vi "test-Coordinate-System-Test5.vi"() -> (3 "All tests passed":bool)   [LabVIEW 2019]
uses:
  <vilib>/Rock Robotics/WPI/ThirdParty/JAS_Junk/TrajLib/VI/CoordAxis_N.vi
  <vilib>/Rock Robotics/WPI/ThirdParty/JAS_Junk/TrajLib/VI/CoordAxis_W.vi
  <vilib>/Rock Robotics/WPI/ThirdParty/JAS_Junk/TrajLib/VI/CoordAxis_U.vi
  <vilib>/Rock Robotics/WPI/ThirdParty/JAS_Junk/TrajLib/VI/CoordSystem_New.vi
  <vilib>/Rock Robotics/WPI/ThirdParty/JAS_Junk/TrajLib/VI/CoordAxis_E.vi
  <vilib>/Rock Robotics/WPI/ThirdParty/JAS_Junk/TrajLib/VI/CoordAxis_D.vi
  <vilib>/Rock Robotics/WPI/ThirdParty/JAS_Junk/TrajLib/Conv_Deg_Radians.vi
  <vilib>/Rock Robotics/WPI/ThirdParty/JAS_Junk/TrajLib/VI/Quaternion_New.vi
  <vilib>/Rock Robotics/WPI/ThirdParty/JAS_Junk/TrajLib/VI/CoordAxis_New.vi
  <vilib>/Rock Robotics/WPI/ThirdParty/JAS_Junk/TrajLib/MatBuilder_Create.vi
  <vilib>/Rock Robotics/WPI/ThirdParty/JAS_Junk/TrajLib/Matrix_AssignBlock.vi
  <vilib>/Rock Robotics/WPI/ThirdParty/JAS_Junk/TrajLib/VI/Rotation3D_Create_RotMatrix.vi
  <vilib>/Rock Robotics/WPI/ThirdParty/JAS_Junk/TrajLib/MatrixHelper_CoerceSize.vi
  <vilib>/Rock Robotics/WPI/ThirdParty/JAS_Junk/TrajLib/VI/Rotation3d_Create_Quaternion.vi
  <vilib>/Rock Robotics/WPI/ThirdParty/JAS_Junk/TrajLib/Matrix_Transpose.vi
  <vilib>/Analysis/baseanly.llb/A x B.vi
  <vilib>/Analysis/baseanly.llb/Real A x B.vi
  <vilib>/Rock Robotics/WPI/ThirdParty/JAS_Junk/TrajLib/Matrix_Ident.vi
  <vilib>/Rock Robotics/WPI/ThirdParty/JAS_Junk/TrajLib/Matrix_IsEqual.vi
  <vilib>/Analysis/baseanly.llb/Determinant.vi
  <vilib>/Analysis/baseanly.llb/Real Determinant.vi
  <vilib>/Rock Robotics/WPI/ThirdParty/JAS_Junk/TrajLib/VI/Quaternion_Normalize.vi
  <vilib>/Rock Robotics/WPI/ThirdParty/JAS_Junk/TrajLib/VI/Quaternion_New_Default.vi
  <vilib>/Analysis/Matrix/Numeric/Conversions/Array To Matrix.vi
  <vilib>/Analysis/Matrix/Numeric/Conversions/Array To Matrix - RA.vi
  <vilib>/Analysis/7linalg.llb/Create Special Matrix.vi
  <vilib>/Analysis/7linalg.llb/Create Special Real Matrix.vi
  <vilib>/Rock Robotics/WPI/ThirdParty/JAS_Junk/TrajLib/Trajectory_Library.lvlib
panel:
  out "Test 4":bool
  out "Test 3":bool
  out "Test 2":bool
  out "Test 1":bool
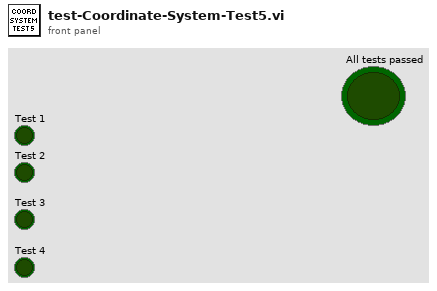
[diagram p1: front panel]
types:
  T1 = typedef "Trajectory_Library.lvlib/TRANSLATION3D.ctl" = cluster{"X":dbl, "Y":dbl, "Z":dbl}
  T2 = typedef "Trajectory_Library.lvlib/ROTATION3D.ctl" = cluster{"Q_quaternion":T3}
  T3 = typedef "Trajectory_Library.lvlib/QUATERNION.ctl" = cluster{"R":dbl, "V":dbl[]}
  T4 = typedef "Trajectory_Library.lvlib/TRANSFORM3D.ctl" = cluster{"TRANSLATION3D":T1, "ROTATION3D":T2, "XF":bool}
  T5 = typedef "Trajectory_Library.lvlib/COORDINATE_SYSTEM.ctl" = cluster{"Rotation":T2}
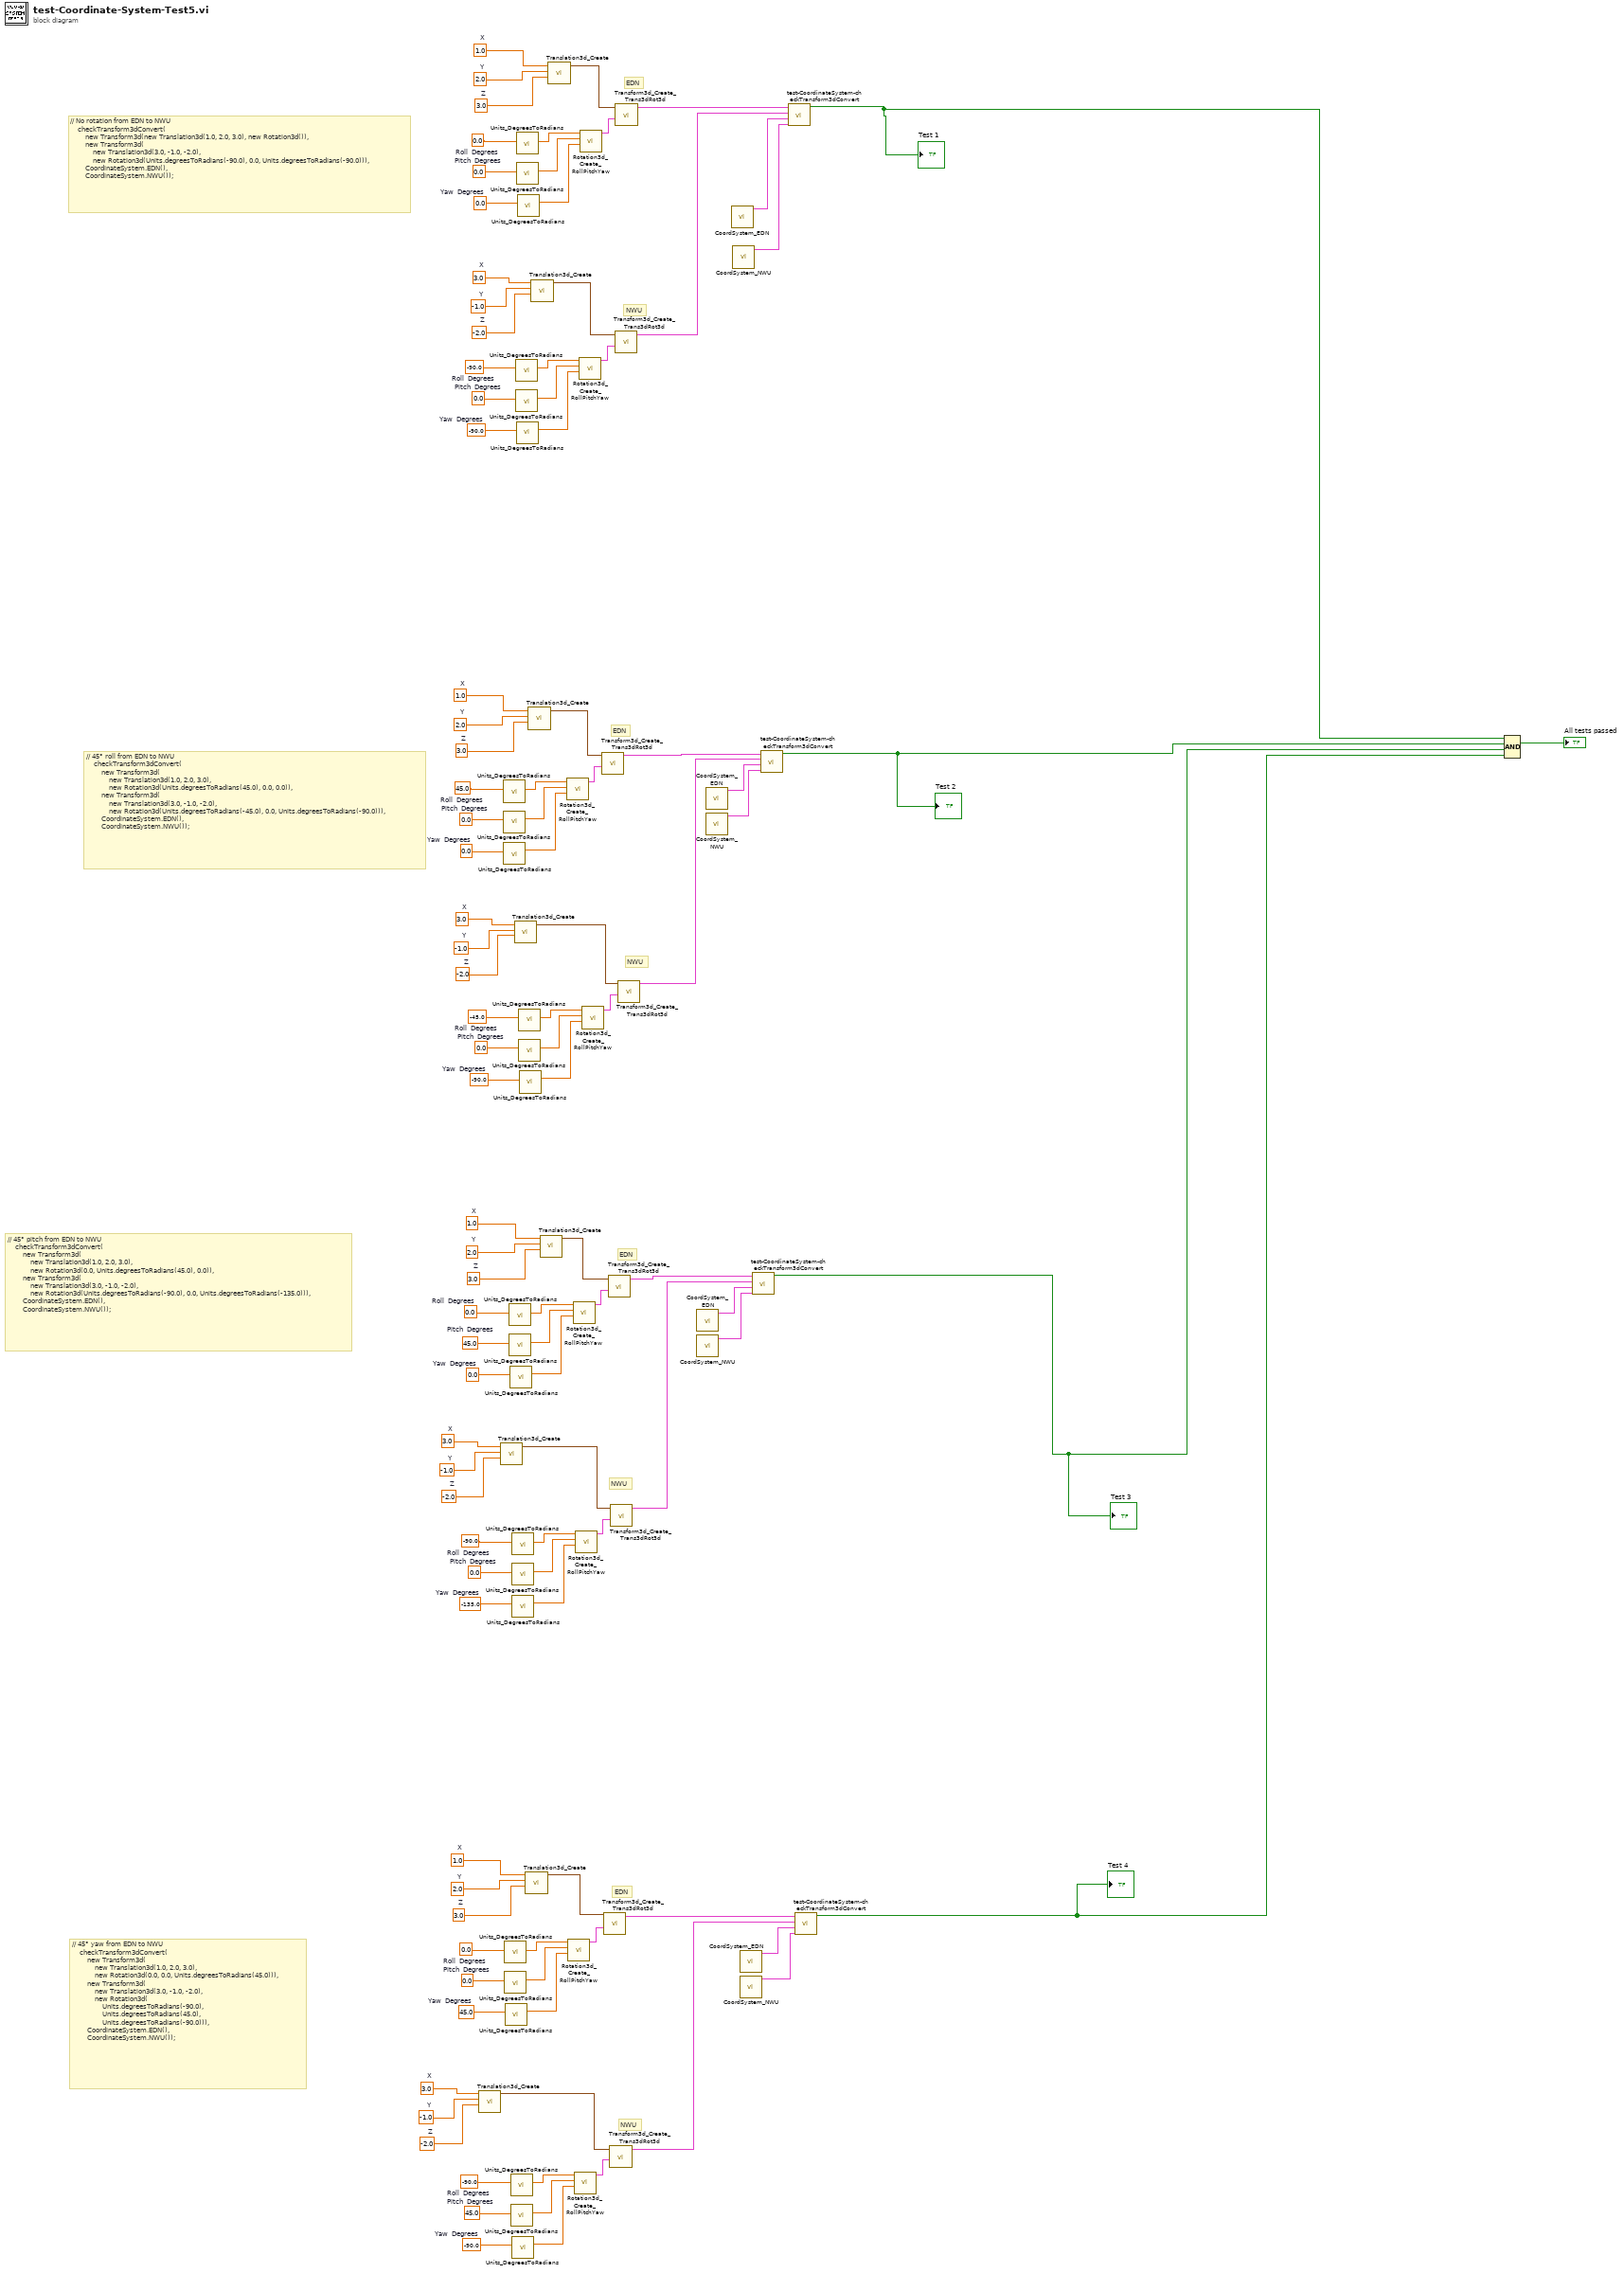
[diagram p0: block diagram]
diagram:
  w8 = 3.0  # X
  w7 = -1.0  # Y
  w6 = -2.0  # Z
  w12 = 3.0  # X
  w11 = -1.0  # Y
  w10 = -2.0  # Z
  w16 = 3.0  # X
  w15 = -1.0  # Y
  w14 = -2.0  # Z
  w24 = 1.0  # X
  w23 = 2.0  # Y
  w22 = 3.0  # Z
  w28 = 1.0  # X
  w27 = 2.0  # Y
  w26 = 3.0  # Z
  w32 = 1.0  # X
  w31 = 2.0  # Y
  w30 = 3.0  # Z
  w53 = -90.0  # Roll  Degrees
  w54 = 45.0  # Pitch  Degrees
  w55 = -90.0  # Yaw  Degrees
  w60 = 0.0  # Roll  Degrees
  w61 = 0.0  # Pitch  Degrees
  w62 = 45.0  # Yaw  Degrees
  w67 = -90.0  # Roll  Degrees
  w68 = 0.0  # Pitch  Degrees
  w69 = -135.0  # Yaw  Degrees
  w74 = 0.0  # Roll  Degrees
  w75 = 45.0  # Pitch  Degrees
  w76 = 0.0  # Yaw  Degrees
  w81 = -45.0  # Roll  Degrees
  w82 = 0.0  # Pitch  Degrees
  w83 = -90.0  # Yaw  Degrees
  w88 = 45.0  # Roll  Degrees
  w89 = 0.0  # Pitch  Degrees
  w90 = 0.0  # Yaw  Degrees
  w20 = 3.0  # X
  w19 = -1.0  # Y
  w18 = -2.0  # Z
  w96 = -90.0  # Roll  Degrees
  w97 = 0.0  # Pitch  Degrees
  w98 = -90.0  # Yaw  Degrees
  w36 = 1.0  # X
  w35 = 2.0  # Y
  w34 = 3.0  # Z
  w103 = 0.0  # Roll  Degrees
  w104 = 0.0  # Pitch  Degrees
  w105 = 0.0  # Yaw  Degrees
  # "// 45° yaw from EDN to NWU\n    checkTransform3dConvert(\n        new Transform3d(\n            new Translation3d(1.0, 2.0, 3.0),\n            new Rotation3d(0.0, 0.0, Units.degreesToRadians(45.0))),\n        new Transform3d(\n            new Translation3d(3.0, -1.0, -2.0),\n            new Rotation3d(\n                Units.degreesToRadians(-90.0),\n                Units.degreesToRadians(45.0),\n                Units.degreesToRadians(-90.0))),\n        CoordinateSystem.EDN(),\n        CoordinateSystem.NWU());"
  # "// No rotation from EDN to NWU\n    checkTransform3dConvert(\n        new Transform3d(new Translation3d(1.0, 2.0, 3.0), new Rotation3d()),\n        new Transform3d(\n            new Translation3d(3.0, -1.0, -2.0),\n            new Rotation3d(Units.degreesToRadians(-90.0), 0.0, Units.degreesToRadians(-90.0))),\n        CoordinateSystem.EDN(),\n        CoordinateSystem.NWU());"
  # "// 45° pitch from EDN to NWU\n    checkTransform3dConvert(\n        new Transform3d(\n            new Translation3d(1.0, 2.0, 3.0),\n            new Rotation3d(0.0, Units.degreesToRadians(45.0), 0.0)),\n        new Transform3d(\n            new Translation3d(3.0, -1.0, -2.0),\n            new Rotation3d(Units.degreesToRadians(-90.0), 0.0, Units.degreesToRadians(-135.0))),\n        CoordinateSystem.EDN(),\n        CoordinateSystem.NWU());"
  # "// 45° roll from EDN to NWU\n    checkTransform3dConvert(\n        new Transform3d(\n            new Translation3d(1.0, 2.0, 3.0),\n            new Rotation3d(Units.degreesToRadians(45.0), 0.0, 0.0)),\n        new Transform3d(\n            new Translation3d(3.0, -1.0, -2.0),\n            new Rotation3d(Units.degreesToRadians(-45.0), 0.0, Units.degreesToRadians(-90.0))),\n        CoordinateSystem.EDN(),\n        CoordinateSystem.NWU());"
  # "NWU"
  # "EDN"
  # "NWU"
  # "EDN"
  # "NWU"
  # "EDN"
  # "NWU"
  # "EDN"
  n1 = call <vilib>:"Translation3d_Create.vi"("Z"=w6, "Y"=w7, "X"=w8) -> ("TRANSLATION3D"=w5:T1)  [unwired: 8 in]
  n2 = call <vilib>:"Translation3d_Create.vi"("Z"=w10, "Y"=w11, "X"=w12) -> ("TRANSLATION3D"=w9:T1)  [unwired: 8 in]
  n3 = call <vilib>:"Units_DegreesToRadians.vi"("Degrees"=w88) -> ("Radians"=w91:dbl)  [unwired: 10 in]
  n4 = call <vilib>:"Units_DegreesToRadians.vi"("Degrees"=w89) -> ("Radians"=w92:dbl)  [unwired: 10 in]
  n5 = call <vilib>:"Units_DegreesToRadians.vi"("Degrees"=w90) -> ("Radians"=w93:dbl)  [unwired: 10 in]
  n6 = call <vilib>:"Units_DegreesToRadians.vi"("Degrees"=w60) -> ("Radians"=w63:dbl)  [unwired: 10 in]
  n7 = call <vilib>:"Units_DegreesToRadians.vi"("Degrees"=w61) -> ("Radians"=w64:dbl)  [unwired: 10 in]
  n8 = call <vilib>:"Units_DegreesToRadians.vi"("Degrees"=w62) -> ("Radians"=w65:dbl)  [unwired: 10 in]
  n9 = call <vilib>:"Units_DegreesToRadians.vi"("Degrees"=w74) -> ("Radians"=w77:dbl)  [unwired: 10 in]
  n10 = call <vilib>:"Units_DegreesToRadians.vi"("Degrees"=w75) -> ("Radians"=w78:dbl)  [unwired: 10 in]
  n11 = call <vilib>:"Units_DegreesToRadians.vi"("Degrees"=w76) -> ("Radians"=w79:dbl)  [unwired: 10 in]
  n12 = call <vilib>:"Units_DegreesToRadians.vi"("Degrees"=w53) -> ("Radians"=w56:dbl)  [unwired: 10 in]
  n13 = call <vilib>:"Units_DegreesToRadians.vi"("Degrees"=w54) -> ("Radians"=w57:dbl)  [unwired: 10 in]
  n14 = call <vilib>:"Units_DegreesToRadians.vi"("Degrees"=w67) -> ("Radians"=w70:dbl)  [unwired: 10 in]
  n15 = call <vilib>:"Units_DegreesToRadians.vi"("Degrees"=w68) -> ("Radians"=w71:dbl)  [unwired: 10 in]
  n16 = call <vilib>:"Units_DegreesToRadians.vi"("Degrees"=w55) -> ("Radians"=w58:dbl)  [unwired: 10 in]
  n17 = call <vilib>:"Units_DegreesToRadians.vi"("Degrees"=w69) -> ("Radians"=w72:dbl)  [unwired: 10 in]
  n18 = call <vilib>:"Translation3d_Create.vi"("Z"=w14, "Y"=w15, "X"=w16) -> ("TRANSLATION3D"=w13:T1)  [unwired: 8 in]
  n19 = call <vilib>:"Units_DegreesToRadians.vi"("Degrees"=w96) -> ("Radians"=w99:dbl)  [unwired: 10 in]
  n20 = call <vilib>:"Units_DegreesToRadians.vi"("Degrees"=w97) -> ("Radians"=w100:dbl)  [unwired: 10 in]
  n21 = call <vilib>:"Units_DegreesToRadians.vi"("Degrees"=w103) -> ("Radians"=w106:dbl)  [unwired: 10 in]
  n22 = call <vilib>:"Units_DegreesToRadians.vi"("Degrees"=w104) -> ("Radians"=w107:dbl)  [unwired: 10 in]
  n23 = call <vilib>:"Units_DegreesToRadians.vi"("Degrees"=w98) -> ("Radians"=w101:dbl)  [unwired: 10 in]
  n24 = call <vilib>:"Units_DegreesToRadians.vi"("Degrees"=w105) -> ("Radians"=w108:dbl)  [unwired: 10 in]
  n25 = call <vilib>:"Units_DegreesToRadians.vi"("Degrees"=w81) -> ("Radians"=w84:dbl)  [unwired: 10 in]
  n26 = call <vilib>:"Units_DegreesToRadians.vi"("Degrees"=w82) -> ("Radians"=w85:dbl)  [unwired: 10 in]
  n27 = call <vilib>:"Units_DegreesToRadians.vi"("Degrees"=w83) -> ("Radians"=w86:dbl)  [unwired: 10 in]
  n28 = call <vilib>:"Translation3d_Create.vi"("Z"=w22, "Y"=w23, "X"=w24) -> ("TRANSLATION3D"=w21:T1)  [unwired: 8 in]
  n29 = call <vilib>:"Translation3d_Create.vi"("Z"=w30, "Y"=w31, "X"=w32) -> ("TRANSLATION3D"=w29:T1)  [unwired: 8 in]
  n30 = call <vilib>:"Translation3d_Create.vi"("Z"=w18, "Y"=w19, "X"=w20) -> ("TRANSLATION3D"=w17:T1)  [unwired: 8 in]
  n31 = call <vilib>:"Translation3d_Create.vi"("Z"=w26, "Y"=w27, "X"=w28) -> ("TRANSLATION3D"=w25:T1)  [unwired: 8 in]
  n32 = call <vilib>:"Translation3d_Create.vi"("Z"=w34, "Y"=w35, "X"=w36) -> ("TRANSLATION3D"=w33:T1)  [unwired: 8 in]
  n33 = call <vilib>:"Rotation3d_Create_RollPitchYaw.vi"("Yaw"=w93, "Pitch"=w92, "Roll"=w91) -> ("Rotation3d"=w94:T2)  [unwired: 8 in]
  n34 = call <vilib>:"Rotation3d_Create_RollPitchYaw.vi"("Yaw"=w65, "Pitch"=w64, "Roll"=w63) -> ("Rotation3d"=w66:T2)  [unwired: 8 in]
  n35 = call <vilib>:"Rotation3d_Create_RollPitchYaw.vi"("Yaw"=w79, "Pitch"=w78, "Roll"=w77) -> ("Rotation3d"=w80:T2)  [unwired: 8 in]
  n36 = call <vilib>:"Rotation3d_Create_RollPitchYaw.vi"("Yaw"=w58, "Pitch"=w57, "Roll"=w56) -> ("Rotation3d"=w59:T2)  [unwired: 8 in]
  n37 = call <vilib>:"Rotation3d_Create_RollPitchYaw.vi"("Yaw"=w72, "Pitch"=w71, "Roll"=w70) -> ("Rotation3d"=w73:T2)  [unwired: 8 in]
  n38 = call <vilib>:"Rotation3d_Create_RollPitchYaw.vi"("Yaw"=w101, "Pitch"=w100, "Roll"=w99) -> ("Rotation3d"=w102:T2)  [unwired: 8 in]
  n39 = call <vilib>:"Rotation3d_Create_RollPitchYaw.vi"("Yaw"=w108, "Pitch"=w107, "Roll"=w106) -> ("Rotation3d"=w109:T2)  [unwired: 8 in]
  n40 = call <vilib>:"Rotation3d_Create_RollPitchYaw.vi"("Yaw"=w86, "Pitch"=w85, "Roll"=w84) -> ("Rotation3d"=w87:T2)  [unwired: 8 in]
  n41 = call <vilib>:"Transform3d_Create_Trans3dRot3d.vi"("Rotation3d"=w94, "Translation3d"=w29) -> ("Transform3d"=w48:T4)  [unwired: 9 in]
  n42 = call <vilib>:"Transform3d_Create_Trans3dRot3d.vi"("Rotation3d"=w66, "Translation3d"=w21) -> ("Transform3d"=w38:T4)  [unwired: 9 in]
  n43 = call <vilib>:"Transform3d_Create_Trans3dRot3d.vi"("Rotation3d"=w80, "Translation3d"=w25) -> ("Transform3d"=w42:T4)  [unwired: 9 in]
  n44 = call <vilib>:"Transform3d_Create_Trans3dRot3d.vi"("Rotation3d"=w59, "Translation3d"=w5) -> ("Transform3d"=w37:T4)  [unwired: 9 in]
  n45 = call <vilib>:"Transform3d_Create_Trans3dRot3d.vi"("Rotation3d"=w73, "Translation3d"=w9) -> ("Transform3d"=w41:T4)  [unwired: 9 in]
  n46 = call <vilib>:"Transform3d_Create_Trans3dRot3d.vi"("Rotation3d"=w102, "Translation3d"=w17) -> ("Transform3d"=w51:T4)  [unwired: 9 in]
  n47 = call <vilib>:"Transform3d_Create_Trans3dRot3d.vi"("Rotation3d"=w109, "Translation3d"=w33) -> ("Transform3d"=w52:T4)  [unwired: 9 in]
  n48 = call <vilib>:"Transform3d_Create_Trans3dRot3d.vi"("Rotation3d"=w87, "Translation3d"=w13) -> ("Transform3d"=w47:T4)  [unwired: 9 in]
  n49 = call <vilib>:"CoordSystem_EDN.vi"() -> ("out Coordinate System"=w44:T5)  [unwired: 10 in, 1 out]
  n50 = call <vilib>:"CoordSystem_NWU.vi"() -> ("out Coordinate System"=w3:T5)  [unwired: 10 in, 1 out]
  n51 = call <vilib>:"CoordSystem_EDN.vi"() -> ("out Coordinate System"=w46:T5)  [unwired: 10 in, 1 out]
  n52 = call <vilib>:"CoordSystem_NWU.vi"() -> ("out Coordinate System"=w2:T5)  [unwired: 10 in, 1 out]
  n53 = call <vilib>:"CoordSystem_EDN.vi"() -> ("out Coordinate System"=w50:T5)  [unwired: 10 in, 1 out]
  n54 = call <vilib>:"CoordSystem_NWU.vi"() -> ("out Coordinate System"=w1:T5)  [unwired: 10 in, 1 out]
  n55 = call <vilib>:"CoordSystem_EDN.vi"() -> ("out Coordinate System"=w40:T5)  [unwired: 10 in, 1 out]
  n56 = call <vilib>:"CoordSystem_NWU.vi"() -> ("out Coordinate System"=w4:T5)  [unwired: 10 in, 1 out]
  n57 = call "test-CoordinateSystem-checkTransform3dConvert.vi"("COORDINATE_SYSTEM_TO"=w3, "COORDINATE_SYSTEM_FROM"=w44, "Transform3D_TO"=w41, "Transform3D_FROM"=w42) -> ("All tests passed"=w43:bool)  [unwired: 7 in]
  "Test 3" <- w43
  n58 = call "test-CoordinateSystem-checkTransform3dConvert.vi"("COORDINATE_SYSTEM_TO"=w2, "COORDINATE_SYSTEM_FROM"=w46, "Transform3D_TO"=w47, "Transform3D_FROM"=w48) -> ("All tests passed"=w45:bool)  [unwired: 7 in]
  "Test 2" <- w45
  n59 = call "test-CoordinateSystem-checkTransform3dConvert.vi"("COORDINATE_SYSTEM_TO"=w1, "COORDINATE_SYSTEM_FROM"=w50, "Transform3D_TO"=w51, "Transform3D_FROM"=w52) -> ("All tests passed"=w49:bool)  [unwired: 7 in]
  "Test 1" <- w49
  n60 = call "test-CoordinateSystem-checkTransform3dConvert.vi"("COORDINATE_SYSTEM_TO"=w4, "COORDINATE_SYSTEM_FROM"=w40, "Transform3D_TO"=w37, "Transform3D_FROM"=w38) -> ("All tests passed"=w39:bool)  [unwired: 7 in]
  "Test 4" <- w39
  n61 = Compound Arithmetic op=AND(w49, w45, w43, w39) -> (→"All tests passed":bool)
